vi "Generate Library Icon.vi"(8 "error in (no error)":errorcluster, 11 "Library":refnum<vi>) -> (0 "error out":errorcluster, 3 "Library out":refnum<vi>)   [LabVIEW 2020, in "New Test Case.lvlib"]
uses:
  New Test Case.lvlib
  <vilib>/LabVIEW Icon API/lv_icon/classes/Icon/Icon.lvclass
  <vilib>/LabVIEW Icon API/API_Rectangle Dimension.ctl
  <vilib>/LabVIEW Icon API/API_Text.ctl
  <vilib>/LabVIEW Icon API/API_Rectangle Colors.ctl
  <vilib>/LabVIEW Icon API/LabVIEW Icon API.lvlib
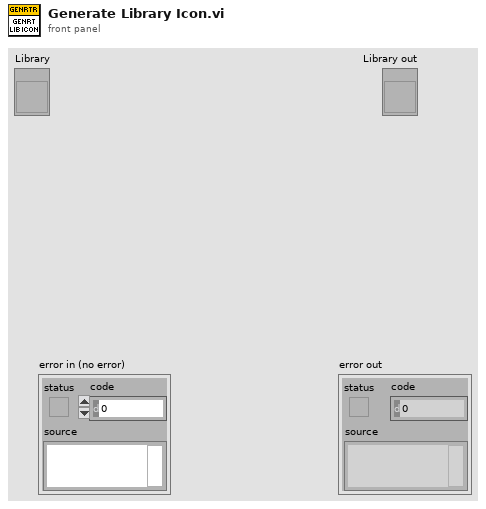
[diagram p1: front panel]
types:
  T1 = typedef "LabVIEW Icon API.lvlib/API_Rectangle Colors.ctl" = cluster{"Border":u32, "Background":u32}
  T2 = typedef "LabVIEW Icon API.lvlib/API_Text.ctl" = cluster{"Line 1 text":string, "Line 2 text":string, "Line 3 text":string, "Line 4 text":string}
  T3 = typedef "LabVIEW Icon API.lvlib/API_Rectangle Dimension.ctl" = cluster{"Width":i16, "Height":i16}
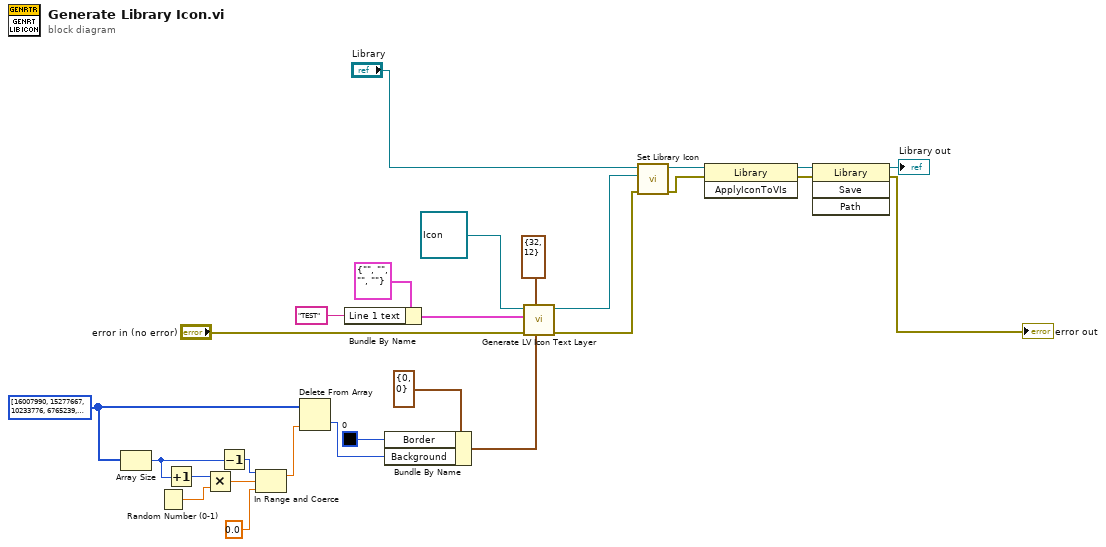
[diagram p0: block diagram]
diagram:
  w16 = u32[] [16007990, 15277667, 10233776, 6765239, 4149685, 2201331, 240116, 48340, 38536, 5025616, 9159498, 13491257, 16771899, 16761095, 16750592, 16733986, 7951688, 10395294, 6323595] ("Array")
  n1 = Array Size(array=w16) -> (size(s)=w10:i32)
  n2 = Random Number (0-1)() -> (number: 0 to 1=w9:dbl)
  n3 = Increment(x=w10) -> (x+1=w11:i32)
  n4 = Multiply(x=w11, y=w9) -> (x*y=w14:dbl)
  n5 = Decrement(x=w10) -> (x-1=w13:i32)
  n6 = In Range and Coerce(upper limit=w13, x=w14, lower limit=0.0) -> (coerced(x)=w8:dbl)  [unwired: 1 out]
  n7 = Delete From Array(array=w16, index=w8) -> (deleted portion=w15:u32)  [unwired: 1 in, 1 out]
  n8 = Bundle By Name(cluster=T2 {"Line 1 text"="", "Line 2 text"="", "Line 3 text"="", "Line 4 text"=""} ("Text"), "Line 1 text"="TEST" ("Overlay Text")) -> (w23:T2)
  n9 = Bundle By Name(cluster=T1 {"Border"=0, "Background"=0} ("Library Color"), "Border"=u32 0 ("Background"), "Background"=w15) -> (w17:T1)
  n10 = call <vilib>:"Generate LV Icon Text Layer.vi"("Rectangle colors (black, white)"=w17, "Rectangle dimension (32,32)"=T3 {"Width"=32, "Height"=12}, "error in (no error)"="error in (no error)", "Text"=w23, "Icon in"=refnum<class "Icon.lvclass"> refnum ("Icon.lvclass in")) -> ("error out"=w20:errorcluster, "Icon out"=w24:refnum<class "Icon.lvclass">)  [unwired: 5 in]
  n11 = call <vilib>:"Set Library Icon.vi"("error in (no error)"=w20, "Icon"=w24, "Library Refnum in"="Library") -> ("error out"=w7:errorcluster, "Library Refnum out"=w2:refnum<vi>)  [unwired: 7 in]
  n12 = invoke class="Library" method="ApplyIconToVIs"(reference=w2, error in=w7) -> (reference out=w1:refnum<vi>, error out=w3:errorcluster)  [unwired: 1 in, 1 out]
  n13 = invoke class="Library" method="Save"(reference=w1, error in=w3) -> (reference out=→"Library out":refnum<vi>, error out=→"error out":errorcluster)  [unwired: 2 in, 2 out]
